vi "string_as_element_name.vi"(11 "result string":string) -> (3 "Array":u8[](array[numeric]))   [LabVIEW 2015, in "BSON_convertors_Library.lvlib"]
uses:
  BSON_convertors_Library.lvlib
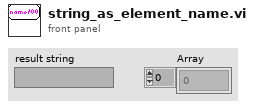
[diagram p1: front panel]
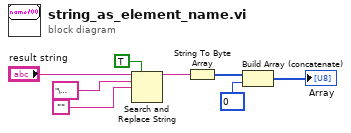
[diagram p0: block diagram]
diagram:
  n1 = Search and Replace String(replace all?=TRUE ("replace all? (F)"), input string="result string", search string="\u0000", replace string="") -> (result string=w1:string)  [unwired: 4 in, 3 out]
  n2 = String To Byte Array(string=w1) -> (unsigned byte array=w6:u8[])
  n3 = Build Array (concatenate)(w6, u8 0) -> (→"Array":u8[])
